vi "WriteToStdOut.vi"(8 "error in (no error)":errorcluster, 10 "Output":string="test output") -> (0 "error out":errorcluster)   [LabVIEW 2014]
uses:
  kernel32.dll
  user32.dll
panel:
  out "lpNumberOfCharsWritten":i32
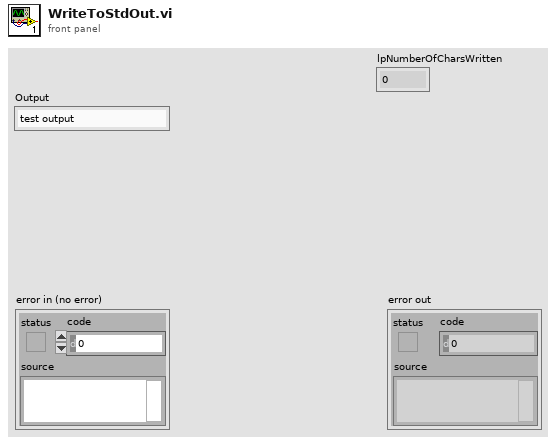
[diagram p1: front panel]
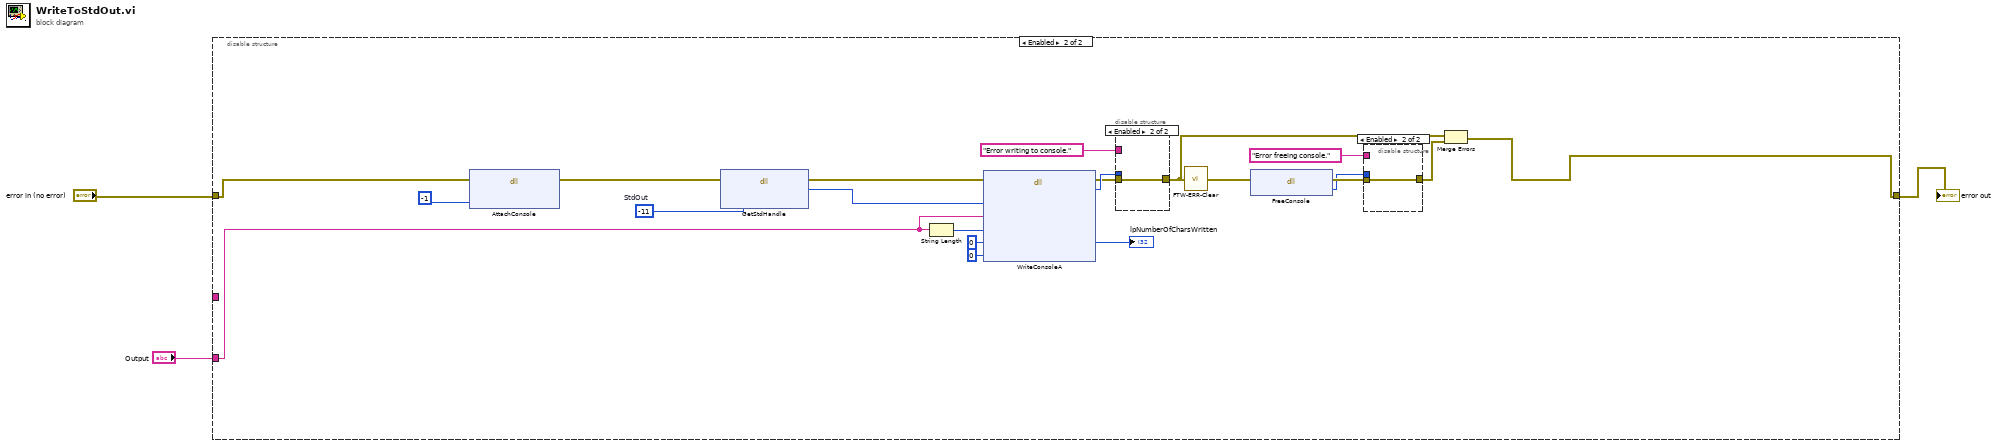
[diagram p0: block diagram]
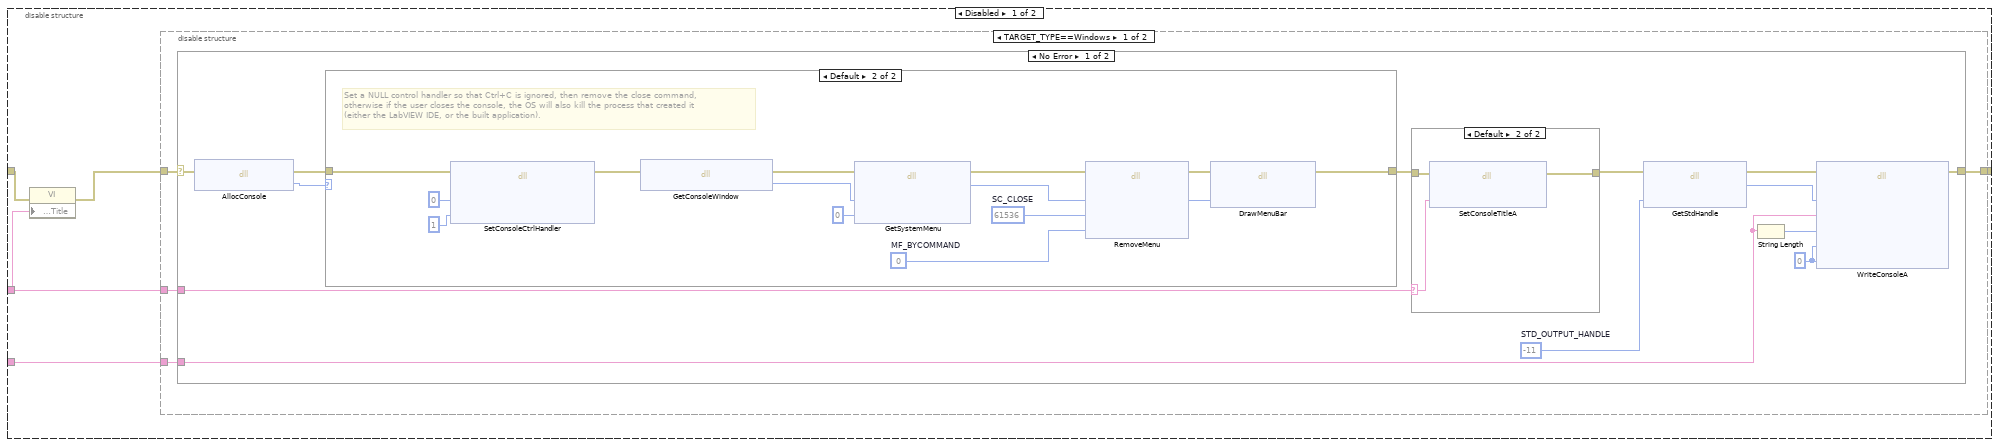
[diagram p2: hidden frame]
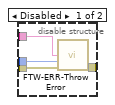
[diagram p7: hidden frame]
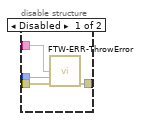
[diagram p8: hidden frame]
diagram:
  n1 = disable-structure shown="Enabled" {
    disable-tunnel: "Output" -> [w8 w61]
    disable-tunnel: [w7 w52] -> w1
    disable-tunnel: "error in (no error)" -> [w6 w60]
    disable-tunnel: _ -> [w4 _]
    frame Disabled {
      n2 = property class="VI"(error in=w6, "Front Panel.Title"=w4) -> (error out=w5:errorcluster)  [unwired: 1 in, 1 out]
      n3 = disable-structure shown="TARGET_TYPE==Windows" {
        disable-tunnel: w5 -> [w11 w46]
        disable-tunnel: [w12 w46] -> w7
        disable-tunnel: w4 -> [w10 _]
        disable-tunnel: w8 -> [w9 _]
        frame condition #0 (active) {
          n4 = case shown="No Error" w11 {
            selector: w11 -> [w25 w45]
            tunnel: [w14 w45] -> w12
            tunnel: w10 -> [w13 _]
            tunnel: w9 -> [w16 _]
            frame No Error {
              w18 = 0 ("lpNumberOfCharsWritten")
              w21 = -11  # STD_OUTPUT_HANDLE
              n5 = dll-call lib="kernel32.dll" fn="AllocConsole"(error in=w25) -> (error out=w23:errorcluster, "return type"=w24:i32)  [unwired: 2 in, 1 out]
              n6 = case shown="Default" w24 {
                tunnel: w23 -> [w30 w31]
                tunnel: [w30 w44] -> w22
                frame 0 {
                  # "Allocation failed, we must already have a console..."
                }
                frame Default {
                  w39 = u32 0  # MF_BYCOMMAND
                  w40 = u32 61536  # SC_CLOSE
                  # "Set a NULL control handler so that Ctrl+C is ignored, then remove the close command,\notherwise if the user closes the console, the OS will also kill the process that created it\n(either the LabVIEW IDE, or the built application)."
                  n7 = dll-call lib="kernel32.dll" fn="SetConsoleCtrlHandler"(error in=w31, "HandlerRoutine"=u32 0, "Add"=1) -> (error out=w34:errorcluster)  [unwired: 2 in, 4 out]
                  n8 = dll-call lib="kernel32.dll" fn="GetConsoleWindow"(error in=w34) -> (error out=w37:errorcluster, "return type"=w43:i32)  [unwired: 2 in, 1 out]
                  n9 = dll-call lib="user32.dll" fn="GetSystemMenu"(error in=w37, "hWnd"=w43, "bRevert"=0) -> (error out=w36:errorcluster, "return type"=w41:i32)  [unwired: 4 in, 1 out]
                  n10 = dll-call lib="user32.dll" fn="RemoveMenu"(error in=w36, "hMenu"=w41, "uPosition"=w40, "uFlags"=w39) -> (error out=w35:errorcluster, "hMenu"=w38:i32)  [unwired: 4 in, 2 out]
                  n11 = dll-call lib="user32.dll" fn="DrawMenuBar"(error in=w35, "hMenu"=w38) -> (error out=w44:errorcluster)  [unwired: 3 in, 2 out]
                }
              }
              n12 = case shown="Default" w13 {
                selector: w13 -> [_ w27]
                tunnel: w22 -> [w26 w29]
                tunnel: [w26 w28] -> w15
                frame "" {
                }
                frame Default {
                  n13 = dll-call lib="kernel32.dll" fn="SetConsoleTitleA"(error in=w29, "lpConsoleTitle"=w27) -> (error out=w28:errorcluster)  [unwired: 2 in, 3 out]
                }
              }
              n14 = dll-call lib="kernel32.dll" fn="GetStdHandle"(error in=w15, "nStdHandle"=w21) -> (error out=w20:errorcluster, "return type"=w19:i32)  [unwired: 3 in, 1 out]
              n15 = String Length(string=w16) -> (length=w17:i32)
              n16 = dll-call lib="kernel32.dll" fn="WriteConsoleA"(error in=w20, "hConsoleOutput"=w19, "lpBuffer"=w16, "numberOfCharsToWrite"=w17, "lpNumberOfCharsWritten"=w18, "lpReserved"=w18) -> (error out=w14:errorcluster)  [unwired: 5 in, 4 out]
            }
            frame Error {
            }
          }
        }
        frame condition #1 {
        }
      }
    }
    frame Enabled {
      w66 = -11  # StdOut
      n17 = dll-call lib="kernel32.dll" fn="AttachConsole"(error in=w60, "arg1"=-1) -> (error out=w47:errorcluster)  [unwired: 4 in, 1 out]
      n18 = dll-call lib="kernel32.dll" fn="GetStdHandle"(error in=w47, "nStdHandle"=w66) -> (error out=w62:errorcluster, "return type"=w63:i32)  [unwired: 3 in, 1 out]
      n19 = String Length(string=w61) -> (length=w64:i32)
      n20 = dll-call lib="kernel32.dll" fn="WriteConsoleA"(error in=w62, "hConsoleOutput"=w63, "lpBuffer"=w61, "numberOfCharsToWrite"=w64, "lpNumberOfCharsWritten"=0, "lpReserved"=0 ("lpNumberOfCharsWritten")) -> (error out=w58:errorcluster, "return type"=w59:i32, "lpNumberOfCharsWritten"=→"lpNumberOfCharsWritten":i32)  [unwired: 5 in, 2 out]
      n21 = disable-structure shown="Enabled" {
        disable-tunnel: w59 -> [w76 _]
        disable-tunnel: w58 -> [w75 w77]
        disable-tunnel: [w74 w77] -> w54
        disable-tunnel: "Error writing to console." ("Error Message") -> [w73 _]
        frame Disabled {
          n22 = call "FTW-ERR-ThrowError.vi"("Error Message"=w73, "Error Code"=w76, "error in"=w75) -> ("error out"=w74:errorcluster)  [unwired: 12 in]
        }
        frame Enabled {
        }
      }
      n23 = call "FTW-ERR-Clear.vi"("error to snuff"=w54) -> ("no error"=w55:errorcluster)
      n24 = dll-call lib="kernel32.dll" fn="FreeConsole"(error in=w55) -> (error out=w57:errorcluster, "Return Value"=w56:i32)  [unwired: 2 in, 1 out]
      n25 = disable-structure shown="Enabled" {
        disable-tunnel: w57 -> [w71 w72]
        disable-tunnel: w56 -> [w70 _]
        disable-tunnel: [w69 w72] -> w53
        disable-tunnel: "Error freeing console." ("Error Message") -> [w68 _]
        frame Disabled {
          n26 = call "FTW-ERR-ThrowError.vi"("Error Message"=w68, "Error Code"=w70, "error in"=w71) -> ("error out"=w69:errorcluster)  [unwired: 12 in]
        }
        frame Enabled {
        }
      }
      n27 = Merge Errors(w54, w53) -> (w52:errorcluster)
    }
  }
  "error out" <- w1
